vi "SVT SNR without Harmonics (Frequency) (1 Ch).vi"(0 "complex spectrum":T7={"complex spectrum response"={"f0"=0.0, "df"=1.0, "complex spectrum"=[]}, "spectrum info"={"channel name"="", "description"="", "x-axis units"=0, "spectral info"={"spectrum type"=enum."Power [Magnitude^2]", "linear/dB"=enum."linear", "window"=0, "window size"=0, "FFT size"=0}, "engineering units"=0, "custom label"="", "dB reference [EU]"=0.0, "peak units"=enum."rms", "weighting filter"=0, "spectral density?"=FALSE, "unit label"="", "spectrum skewed?"=FALSE, "complimentary spectrum units"=enum."none"}} {"spectrum info"."x-axis units" items=["Time (s)"=0, "Frequency-CB (Hz)"=1, "Frequency-CPB (Hz)"=1248, "Frequency-Arbitrary (Hz)"=2357, "Quefrency (s)"=2, "Revolutions (rev)"=3, "Order"=4, "Speed (RPM)"=11, "Speed (rad/s)"=21, "Index"=65535]; "spectrum info"."weighting filter" items=["Linear", "A-weighting", "B-weighting", "C-weighting", "ITU-R 468-4", "Dolby", "CCITT", "C-message", "Wb", "Wc", "Wd", "We", "Wf", "Wh", "Wj", "Wk", "Wm", "AES17 20 kHz lowpass", "AES17 40 kHz lowpass", "AES17 20 kHz highpass", "AES17 40 kHz highpass"]; "spectrum info"."dB reference [EU]" format="%.2f"; "spectrum info"."engineering units" items=["custom..."=0, "V"=1, "A"=21, "C"=30, "pC"=31, "s"=32, "-"=29, "Pa"=2, "N"=20, "g"=3, "m/s^2"=4, "m/s"=5, "m"=6, "mm/s"=12, "mm"=13, "micron/s"=14, "micron"=15, "in/s^2"=7, "in/s"=8, "in"=9, "mil/s"=10, "mil"=11, "rad/s^2"=16, "rad/s"=17, "rad"=18, "deg/s^2"=26, "deg/s"=27, "deg"=28, "RPM"=22, "cycle/s^2"=23, "Hz"=24, "cycle"=25, "strain"=19]; "spectrum info"."spectral info"."window" items=["None "=0, "Hanning"=1, "Hamming"=2, "Blackman-Harris"=3, "Exact Blackman"=4, "Blackman"=5, "Flat Top"=6, "4 Term B-Harris "=7, "7 Term B-Harris"=8, "Low Sidelobe"=9, "Force - Exponential"=10, "Gaussian"=62]; "complex spectrum response"."complex spectrum" format="%.2f"; "complex spectrum response"."df" format="%.2f"; "complex spectrum response"."f0" format="%.2f"}, 2 "frequency range":T10={"start frequency"=-1.0, "stop frequency"=-1.0} {"stop frequency" format="%.2f"; "start frequency" format="%.2f"}, 3 "advanced span [Hz]":dbl=-1.0 format="%.2f", 4 "maximum harmonic":i32=-1, 5 "error in (no error)":errorcluster, 6 "desired units":T9, 9 "expected fundamental frequency [Hz]":dbl=-1.0 format="%.2f") -> (11 "detected fundamental\nfrequency [Hz]":dbl format="%.2f", 12 "unit labels":T8, 13 "detected fundamental\namplitude":dbl format="%.2f", 14 "complex spectrum":T7={"complex spectrum response"={"f0"=0.0, "df"=1.0, "complex spectrum"=[]}, "spectrum info"={"channel name"="", "description"="", "x-axis units"=0, "spectral info"={"spectrum type"=enum."Power [Magnitude^2]", "linear/dB"=enum."linear", "window"=0, "window size"=0, "FFT size"=0}, "engineering units"=0, "custom label"="", "dB reference [EU]"=0.0, "peak units"=enum."rms", "weighting filter"=0, "spectral density?"=FALSE, "unit label"="", "spectrum skewed?"=FALSE, "complimentary spectrum units"=enum."none"}} {"spectrum info"."x-axis units" items=["Time (s)"=0, "Frequency-CB (Hz)"=1, "Frequency-CPB (Hz)"=1248, "Frequency-Arbitrary (Hz)"=2357, "Quefrency (s)"=2, "Revolutions (rev)"=3, "Order"=4, "Speed (RPM)"=11, "Speed (rad/s)"=21, "Index"=65535]; "spectrum info"."weighting filter" items=["Linear", "A-weighting", "B-weighting", "C-weighting", "ITU-R 468-4", "Dolby", "CCITT", "C-message", "Wb", "Wc", "Wd", "We", "Wf", "Wh", "Wj", "Wk", "Wm", "AES17 20 kHz lowpass", "AES17 40 kHz lowpass", "AES17 20 kHz highpass", "AES17 40 kHz highpass"]; "spectrum info"."dB reference [EU]" format="%.2f"; "spectrum info"."engineering units" items=["custom..."=0, "V"=1, "A"=21, "C"=30, "pC"=31, "s"=32, "-"=29, "Pa"=2, "N"=20, "g"=3, "m/s^2"=4, "m/s"=5, "m"=6, "mm/s"=12, "mm"=13, "micron/s"=14, "micron"=15, "in/s^2"=7, "in/s"=8, "in"=9, "mil/s"=10, "mil"=11, "rad/s^2"=16, "rad/s"=17, "rad"=18, "deg/s^2"=26, "deg/s"=27, "deg"=28, "RPM"=22, "cycle/s^2"=23, "Hz"=24, "cycle"=25, "strain"=19]; "spectrum info"."spectral info"."window" items=["None "=0, "Hanning"=1, "Hamming"=2, "Blackman-Harris"=3, "Exact Blackman"=4, "Blackman"=5, "Flat Top"=6, "4 Term B-Harris "=7, "7 Term B-Harris"=8, "Low Sidelobe"=9, "Force - Exponential"=10, "Gaussian"=62]; "complex spectrum response"."complex spectrum" format="%.2f"; "complex spectrum response"."df" format="%.2f"; "complex spectrum response"."f0" format="%.2f"}, 16 "SNR (without harmonics)":dbl format="%.2f", 17 "SINAD":dbl format="%.2f", 18 "THD":dbl format="%.2f", 19 "error out":errorcluster)   [LabVIEW 2017, in "SoundVib_Distortion.lvlib"]
doc: "Performs a signal and noise analysis, including measuring the fundamental tone, and returns the detected fundamental frequency, detected fundamental amplitude, and signal-to-noise ratio (SNR) (without harmonics). The SNR measurement excludes harmonics of the fundamental frequency. Wire data to the <B>scaled signal [EU]</B> input to determine the polymorphic instance to use or manually select the instance.\n\nThe following formula calculates SNR:\n\nSNR = F / N\n\nwhere F is the fundamental tone RMS level and N is the noise RMS."
uses:
  <vilib>/addons/Sound and Vibration/svt_Distortion/SoundVib_Distortion.lvlib
  <vilib>/addons/_NISVFA/_Shared subVIs/Controls/svc_Spectrum Info.ctl
  <vilib>/addons/_NISVFA/_Shared subVIs/Controls/svc_X-Axis Units.ctl
  <vilib>/addons/_NISVFA/_Shared subVIs/Controls/svc_Spectrum Type.ctl
  <vilib>/addons/_NISVFA/_Shared subVIs/Controls/svc_Engineering Units Text Ring.ctl
  <vilib>/addons/_NISVFA/_Shared subVIs/Controls/svc_Weighting Filter Text Ring.ctl
  <vilib>/addons/_NISVFA/_Shared subVIs/Controls/svc_Complimentary Spectrum Units.ctl
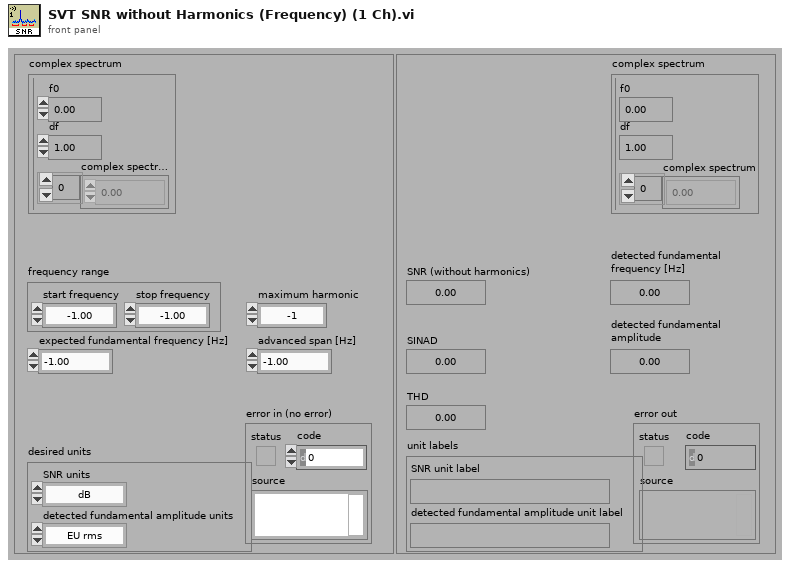
[diagram p1: front panel]
types:
  T1 = typedef "svc_Spectrum Info.ctl" = cluster{"channel name":string, "description":string, "x-axis units":T2, "spectral info":cluster{"spectrum type":T3, "linear/dB":enum16{"linear", "dB"}, "window":u16, "window size":i32, "FFT size":i32}, "engineering units":T4, "custom label":string, "dB reference [EU]":dbl, "peak units":enum16{"rms", "peak", "peak-peak"}, "weighting filter":T5, "spectral density?":bool, "unit label":string, "spectrum skewed?":bool, "complimentary spectrum units":T6}
  T2 = typedef "svc_X-Axis Units.ctl" = u16
  T3 = typedef "svc_Spectrum Type.ctl" = enum16{"FFT Spectrum [complex]", "Amplitude [Magnitude]", "Power [Magnitude^2]", "Cross Spectrum [complex]", "Frequency Response [Complex]"}
  T4 = typedef "svc_Engineering Units Text Ring.ctl" = u16
  T5 = typedef "svc_Weighting Filter Text Ring.ctl" = u16
  T6 = typedef "svc_Complimentary Spectrum Units.ctl" = enum16{"none", "radians", "degrees", "cycles", "imaginary"}
  T7 = cluster{"complex spectrum response":cluster{"f0":dbl, "df":dbl, "complex spectrum":cdb[]}, "spectrum info":T1}
  T8 = cluster{"SNR unit label":string, "detected fundamental amplitude unit label":string}
  T9 = cluster{"SNR units":enum16{"dB", "linear ratio", "%"}, "detected fundamental amplitude units":enum16{"EU rms", "EU peak", "EU peak-peak"}}
  T10 = cluster{"start frequency":dbl, "stop frequency":dbl}
  T11 = cluster{"SINAD [ratio]":dbl, "THD+N [ratio]":dbl, "THD":dbl}
  T12 = cluster{"total":dbl, "fundamental":dbl, "noise and harmonics":dbl, "harmonic energy":dbl, "noise":dbl}
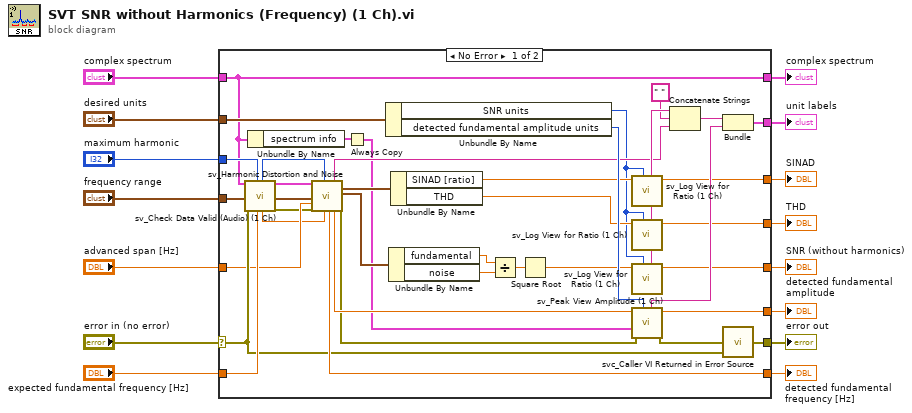
[diagram p0: block diagram]
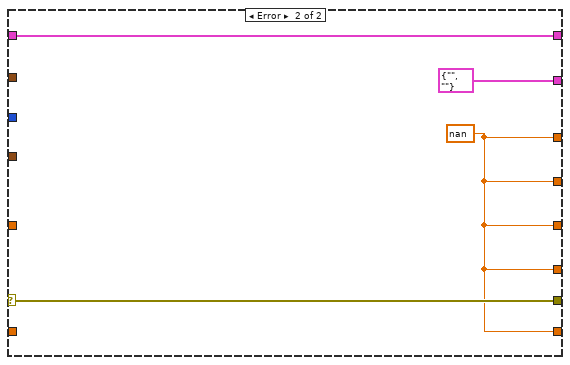
[diagram p2: hidden frame]
diagram:
  n1 = case shown="No Error" "error in (no error)" {
    selector: "error in (no error)" -> [w41 w58]
    tunnel: "expected fundamental frequency [Hz]" -> [w47 _]
    tunnel: [w51 w58] -> w15
    tunnel: [w38 w56] -> w14
    tunnel: [w53 w56] -> w13
    tunnel: [w43 w56] -> w12
    tunnel: "desired units" -> [w54 _]
    tunnel: [w52 cluster{string, string} {"", ""}] -> w10
    tunnel: "frequency range" -> [w46 _]
    tunnel: "advanced span [Hz]" -> [w34 _]
    tunnel: [w37 w56] -> w5
    tunnel: [w36 w56] -> w4
    tunnel: "maximum harmonic" -> [w21 _]
    tunnel: [w16 w55] -> w2
    tunnel: "complex spectrum" -> [w16 w55]
    frame No Error {
      n2 = call <vilib>:"sv_Check Data Valid (Audio) (1 Ch).vi"("complex spectrum"=w16, "frequency range in"=w46, "error in (no error)"=w41, "maximum harmonic"=w21, "expected fundamental frequency [Hz]"=w47) -> ("dup maximum harmonic"=w20:i32, "dup expected fundamental frequency [Hz]"=w28:dbl, "complex spectrum"=w17:T7, "frequency range out"=w35:T10, "error out"=w29:errorcluster)  [unwired: 7 in, 3 out]
      n3 = Unbundle By Name(w16) -> ("spectrum info"=w45:T1)
      n4 = call <vilib>:"sv_Harmonic Distortion and Noise.vi"("complex spectrum"=w17, "frequency range"=w35, "advanced span [Hz]"=w34, "error in"=w29, "maximum harmonic"=w20, "approx. fund. freq. (optional)"=w28) -> ("detected fundamental frequency"=w43:dbl, "frequency range string"=w33:string, "detected amplitude"=w42:dbl, "distortion measurements"=w32:T11, "energy"=w27:T12, "error out"=w18:errorcluster)  [unwired: 6 in, 2 out]
      n5 = Always Copy(1:w45) -> (0:w19:T1)
      n6 = Unbundle By Name(w54) -> ("SNR units"=w24:enum16{"dB", "linear ratio", "%"}, "detected fundamental amplitude units"=w40:enum16{"EU rms", "EU peak", "EU peak-peak"})
      n7 = Unbundle By Name(w27) -> ("fundamental"=w26:dbl, "noise"=w25:dbl)
      n8 = Unbundle By Name(w32) -> ("SINAD [ratio]"=w30:dbl, "THD"=w31:dbl)
      n9 = Divide(x=w26, y=w25) -> (x/y=w23:dbl)
      n10 = Square Root(x=w23) -> (sqrt(x)=w22:dbl)
      n11 = call <vilib>:"sv_Log View for Ratio (1 Ch).vi"("ratio units"=w24, "linear ratio"=w30) -> ("converted ratio"=w37:dbl)  [unwired: 7 in, 2 out]
      n12 = call <vilib>:"sv_Log View for Ratio (1 Ch).vi"("ratio units"=w24, "linear ratio"=w31) -> ("converted ratio"=w36:dbl)  [unwired: 7 in, 2 out]
      n13 = call <vilib>:"sv_Log View for Ratio (1 Ch).vi"("ratio units"=w24, "linear ratio"=w22) -> ("converted ratio"=w38:dbl, "unit label"=w49:string)  [unwired: 7 in, 1 out]
      n14 = call <vilib>:"sv_Peak View Amplitude (1 Ch).vi"("peak units"=w40, "error in (no error)"=w18, "spectrum info"=w19, "peak amplitude [EU pk]"=w42) -> ("error out"=w44:errorcluster, "converted peak amplitude"=w53:dbl, "unit label"=w39:string)  [unwired: 5 in]
      n15 = Concatenate Strings(w49, " " ("string"), w33) -> (w50:string)
      n16 = Bundle(w50, "unit label"=w39) -> (w52:cluster{string, "unit label":string})  [unwired: 1 in]
      n17 = call <vilib>:"svc_Caller VI Returned in Error Source.vi"("warning input to caller"=w41, "error in (no error)"=w44) -> ("error out"=w51:errorcluster)  [unwired: 3 in]
    }
    frame Error {
      w56 = nan ("SINAD")
    }
  }
  "error out" <- w15
  "SNR (without harmonics)" <- w14
  "unit labels" <- w10
  "detected fundamental\nfrequency [Hz]" <- w12
  "detected fundamental\namplitude" <- w13
  "complex spectrum" <- w2
  "SINAD" <- w5
  "THD" <- w4
